vi "Make_Mirror_Pattern_V1.vi"(0 "Mirror Modes In":T1, 2 "Flat On?":bool, 7 "Flat File In":dbl[](array[numeric]), 11 "Mirror Modes Array":dbl[][](array[numeric])) -> (8 "Pixel Value U (-1 to 1)":dbl[](array[numeric]))   [LabVIEW 2014]
uses:
  Controls/MirrorModes.ctl
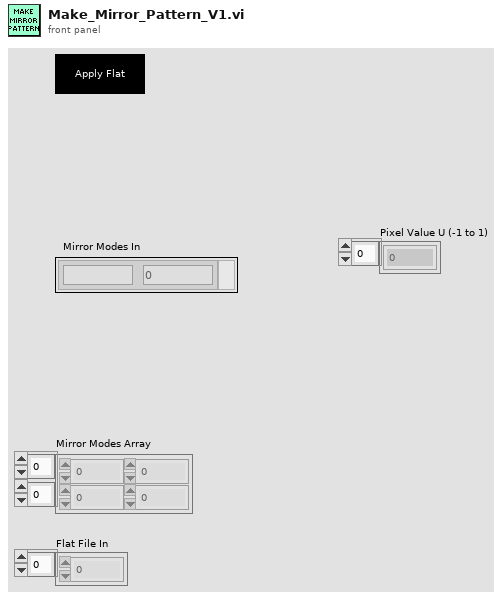
[diagram p1: front panel]
types:
  T1 = typedef "MirrorModes.ctl" = cluster{"Mode":string, "Amplitude":dbl}[]
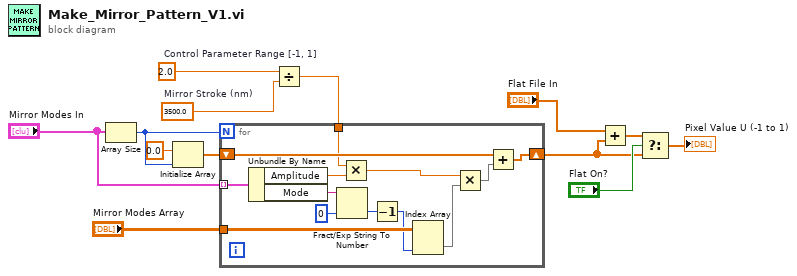
[diagram p0: block diagram]
diagram:
  w11 = 3500.0  # Mirror Stroke (nm)
  w10 = 2.0  # Control Parameter Range [-1, 1]
  n1 = Array Size(array="Mirror Modes In") -> (size(s)=w12:i32)
  n2 = Initialize Array(0.0 ("element"), w12) -> (w2:dbl[])
  n3 = Divide(x=w10, y=w11) -> (x/y=w9:dbl)
  n4 = for {
    N: w12 -> [_]
    tunnel: "Mirror Modes In" -> [w26] mode=indexing
    shift-right: [w19] -> w3
    shift-left: w2 -> [w20]
    tunnel: "Mirror Modes Array" -> [w22]
    tunnel: w9 -> [w16]
    n5 = Unbundle By Name(w26) -> ("Amplitude"=w17:dbl, "Mode"=w24:string)
    n6 = Fract/Exp String To Number(string=w24, default (0 dbl)=0) -> (number=w23:i32)  [unwired: 2 in, 1 out]
    n7 = Multiply(x=w16, y=w17) -> (x*y=w14:dbl)
    n8 = Decrement(x=w23) -> (x-1=w21:i32)
    n9 = Index Array(array=w22, index (col)=w21) -> (element=w15:dbl[])  [unwired: 1 in]
    n10 = Multiply(x=w14, y=w15) -> (x*y=w18:dbl[])
    n11 = Add(x=w20, y=w18) -> (x+y=w19:dbl[])
  }
  n12 = Add(x="Flat File In", y=w3) -> (x+y=w8:dbl[])
  n13 = Select(t=w8, s="Flat On?", f=w3) -> (s? t:f=→"Pixel Value U (-1 to 1)":dbl[])
